vi "LVCAM Receive.vi"(11 "Actor in":refnum<class "Actor.lvclass">) -> (0 "error out":errorcluster, 2 "Msg":refnum<class "Msg.lvclass">)   [LabVIEW 2021, in "LVCAM.lvlib" / "Actor.lvclass"]
uses:
  Actor.lvclass
  Msg/Msg.lvclass
  Actor.lvclass/Actor.ctl
  Msgs/LVCAM Nest Destroyed/LVCAM Nest Destroyed Msg/LVCAM Nest Destroyed Msg.lvclass
  C:/PPLs/LabVIEW-Composed-Actor-Model-LVCAM/LabVIEW-Composed-Actor-Model-LVCAM/LVCAM/LVCAM/Msg/Msg.lvclass
  Msgs/LVCAM Destroy Self/LVCAM Destroy Self Msg/LVCAM Destroy Self Msg.lvclass
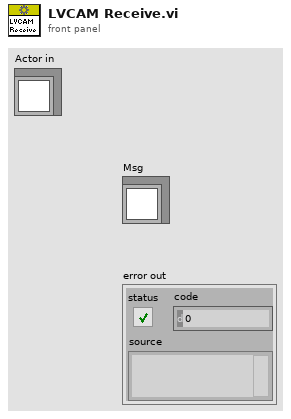
[diagram p1: front panel]
types:
  T1 = typedef "LVCAM.lvlib/Actor.lvclass/State.ctl" = enum16{"Msging", "Destroying", "Destroyed"}
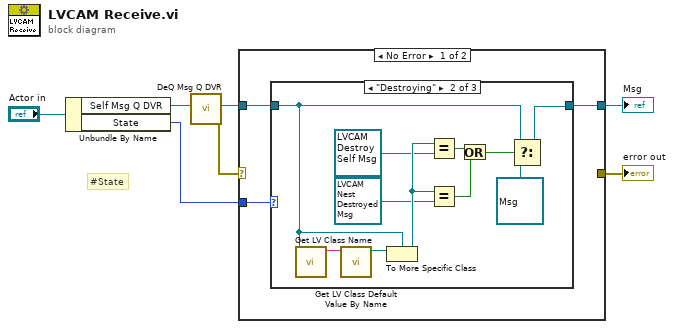
[diagram p0: block diagram]
diagram:
  # "#State"
  n1 = Unbundle By Name("Actor in") -> ("Self Msg Q DVR"=w5:refnum<data-value>, "State"=w7:T1)
  n2 = call "DeQ Msg Q DVR.vi"("Msg Q DVR"=w5) -> ("error out"=w4:errorcluster, "Msg"=w1:refnum<class "Msg.lvclass">)  [unwired: 9 in]
  n3 = case shown="No Error" w4 {
    selector: w4 -> [_ w24]
    tunnel: w7 -> [w10 _]
    tunnel: [_ w24] -> w6
    tunnel: [w9 _] -> w2
    tunnel: w1 -> [w8 _]
    frame No Error {
      n4 = case shown="\"Destroying\"" w10 {
        tunnel: [w11 w13 w23] -> w9
        tunnel: w8 -> [w11 w12 w23]
        frame "Msging" {
        }
        frame "Destroying" {
          n5 = call <vilib>:"Get LV Class Name.vi"("object"=w12) -> ("class name"=w22:string)  [unwired: 9 in, 1 out]
          n6 = call <vilib>:"Get LV Class Default Value By Name.vi"("class name"=w22) -> ("object"=w21:refnum<class>)  [unwired: 9 in, 1 out]
          n7 = To More Specific Class(target class=w12, reference=w21) -> (specific class reference=w19:refnum<class "Msg.lvclass">)  [unwired: 1 in, 1 out]
          n8 = Equal?(x=w19, y=refnum<class "LVCAM Destroy Self Msg.lvclass"> refnum ("LVCAM Destroy Self.lvlib:LVCAM Destroy Self Msg.lvclass")) -> (x = y?=w20:bool)
          n9 = Equal?(x=w19, y=refnum<class "LVCAM Nest Destroyed Msg.lvclass"> refnum ("LVCAM Nest Destroyed.lvlib:LVCAM Nest Destroyed Msg.lvclass")) -> (x = y?=w17:bool)
          n10 = Or(x=w20, y=w17) -> (x .or. y?=w15:bool)
          n11 = Select(t=w12, s=w15, f=refnum<class "Msg.lvclass"> refnum) -> (s? t:f=w13:refnum<class "Msg.lvclass">)
        }
        frame "Destroyed" {
        }
      }
    }
    frame Error {
      # "#LVCAM Error"
    }
  }
  "Msg" <- w2
  "error out" <- w6
